vi "WriteDO.vi"(8 "error in (no error)":errorcluster, 10 "gRPCid":T5, 11 "DIOSessions In":T1={"Array of DI Sessions"=[], "Array of DO Sessions"=[], "Stream ReadDI"={"gRPCid ReadDI"=0, "DISessionName"="", "Stream Status ReadDI"=FALSE, "Async Stop ReadDI Queue"=refnum, "DI Task"="", "ms to wait"=500}}) -> (0 "error out":errorcluster, 3 "DIOSessions Out":T1={"Array of DI Sessions"=[], "Array of DO Sessions"=[], "Stream ReadDI"={"gRPCid ReadDI"=0, "DISessionName"="", "Stream Status ReadDI"=FALSE, "Async Stop ReadDI Queue"=refnum, "DI Task"="", "ms to wait"=500}})   [LabVIEW 2019, in "ctet_dio_User Library.lvlib"]
uses:
  ctet_dio_User Library.lvlib
  Servers/ctet_dio/gRPC lvSupport/Server API/typeDefs/grpcId.ctl
  Types/DIOSessions.ctl
  Types/DISession.ctl
  Types/DOSession.ctl
  Types/StreamReadDI.ctl
  Servers/ctet_dio/ctet_dio Class/RPC Messages/measurementservice_WriteDOResponse/measurementservice_WriteDOResponse_Data.ctl
  Servers/ctet_dio/ctet_dio Class/RPC Messages/measurementservice_ErrorOut/measurementservice_ErrorOut_Data.ctl
  <vilib>/DAQmx/write.llb/DAQmx Write (Digital 1D Bool NChan 1Samp 1Line).vi
  <vilib>/DAQmx/miscellaneous.llb/DAQmx Fill In Error Info.vi
  Servers/ctet_dio/ctet_dio Class/ctet_dio.lvclass
  Servers/ctet_dio/gRPC lvSupport/gprc-lvsupport.lvlib
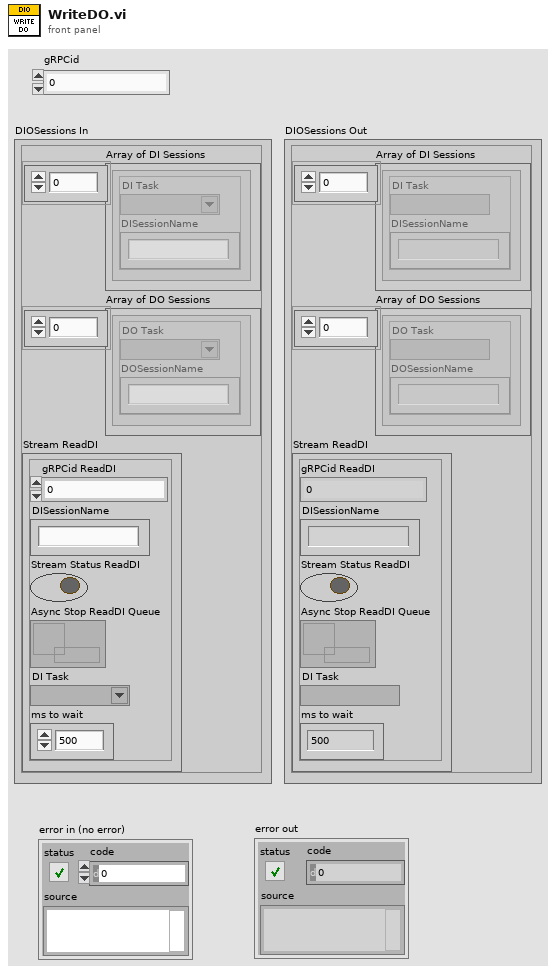
[diagram p1: front panel]
types:
  T1 = typedef "ctet_dio_User Library.lvlib/DIOSessions.ctl" = cluster{"Array of DI Sessions":T2[], "Array of DO Sessions":T3[], "Stream ReadDI":T4}
  T2 = typedef "ctet_dio_User Library.lvlib/DISession.ctl" = cluster{"DI Task":refnum<k21>, "DISessionName":string}
  T3 = typedef "ctet_dio_User Library.lvlib/DOSession.ctl" = cluster{"DO Task":refnum<k21>, "DOSessionName":string}
  T4 = typedef "ctet_dio_User Library.lvlib/StreamReadDI.ctl" = cluster{"gRPCid ReadDI":T5, "DISessionName":string, "Stream Status ReadDI":bool, "Async Stop ReadDI Queue":refnum<queue>, "DI Task":refnum<k21>, "ms to wait":u32}
  T5 = typedef "ctet_dio.lvlib/gprc-lvsupport.lvlib/grpcId.ctl" = u64
  T6 = typedef "ctet_dio.lvlib/ctet_dio.lvclass/measurementservice_ErrorOut_Data.ctl" = cluster{"errCode":i64, "errMessage":string}
  T7 = typedef "ctet_dio.lvlib/ctet_dio.lvclass/measurementservice_WriteDOResponse_Data.ctl" = cluster{"DOSessionName":string, "DOData":bool[], "error":T6}
  T8 = typedef "ctet_dio.lvlib/ctet_dio.lvclass/measurementservice_WriteDORequest_Data.ctl" = cluster{"DOSessionName":string, "DOData":bool[]}
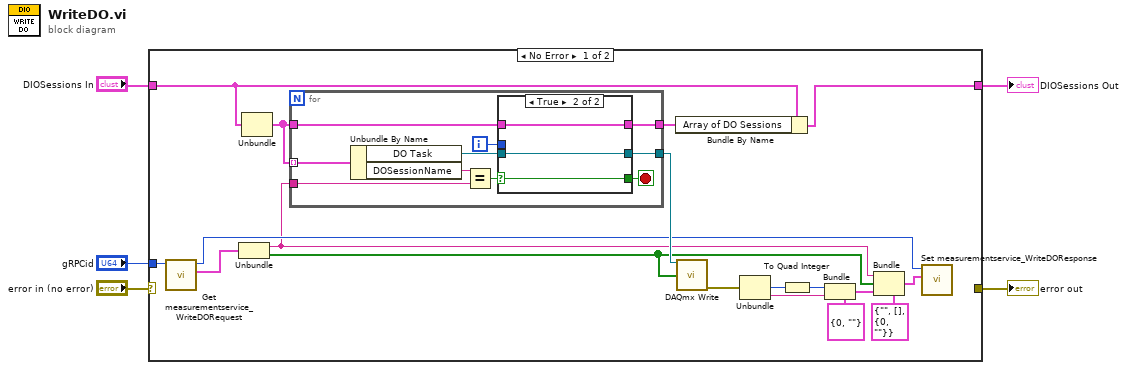
[diagram p0: block diagram]
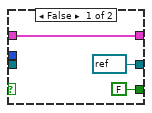
[diagram p2: hidden frame]
diagram:
  n1 = case shown="No Error" "error in (no error)" {
    selector: "error in (no error)" -> [_ w41]
    tunnel: [_ w41] -> w5
    tunnel: "gRPCid" -> [w20 _]
    tunnel: "DIOSessions In" -> [w7 w40]
    tunnel: [w6 w40] -> w1
    frame No Error {
      n2 = call "Get measurementservice_WriteDORequest.vi"("gRPCid"=w20) -> ("Message Data"=w19:T8, "gRPCid out"=w10:T5)  [unwired: 8 in, 1 out]
      n3 = Unbundle(w19) -> ("DOSessionName"=w9:string, "DOData"=w8:bool[])
      n4 = Unbundle(w7) -> ("Array of DO Sessions"=w14:T3[])  [unwired: 2 out]
      n5 = for {
        tunnel: w14 -> [w28] mode=indexing
        tunnel: w9 -> [w33]
        tunnel: [w29] -> w13
        tunnel: w14 -> [w27]
        tunnel: [w26] -> w12
        i -> [w24]
        stop <- w31 stop-if-true
        n6 = Unbundle By Name(w28) -> ("DO Task"=w30:refnum<k21>, "DOSessionName"=w25:string)
        n7 = Equal?(x=w25, y=w33) -> (x = y?=w32:bool)
        n8 = case shown="True" w32 {
          selector: w32 -> [_ w39]
          tunnel: [FALSE w39] -> w31
          tunnel: w30 -> [_ w37]
          tunnel: [refnum<k21> refnum ("DI Task") w37] -> w29
          tunnel: w27 -> [w34 w38]
          tunnel: [w34 w38] -> w26
          tunnel: w24 -> [_ _]
          frame False {
          }
          frame True {
          }
        }
      }
      n9 = Bundle By Name(cluster=w7, "Array of DO Sessions"=w12) -> (w6:T1)
      n10 = call-poly <vilib>:"DAQmx Write.vi"("task/channels in"=w13, "data"=w8) -> ("error out"=w11:errorcluster)  [unwired: 11 in, 2 out]
      n11 = Unbundle(w11) -> ("code"=w22:i32, "source"=w23:string)  [unwired: 1 out]
      n12 = To Quad Integer(1:w22) -> (0:w21:i64)
      n13 = Bundle(cluster=T6 {"errCode"=0, "errMessage"=""} ("error"), "errCode"=w21, "errMessage"=w23) -> (w15:T6)
      n14 = Bundle(cluster=T7 {"DOSessionName"="", "DOData"=[], "error"={"errCode"=0, "errMessage"=""}} ("measurementservice_WriteDOResponse_Data"), "DOSessionName"=w9, "DOData"=w8, "error"=w15) -> (w18:T7)
      n15 = call "Set measurementservice_WriteDOResponse.vi"("Message Data"=w18, "gRPCid"=w10) -> ()  [unwired: 9 in, 1 out]
    }
    frame Error {
    }
  }
  "error out" <- w5
  "DIOSessions Out" <- w1
